vi "Kaelus PIM Config Load Instruments.vi"(7 "Tree":refnum<vi>, 8 "error in (no error)":errorcluster, 9 "Interface":T1, 10 "Port":u16=3388, 11 "IP":string="localhost" caption="Machine Location (IP / Fully Qualified Domain Name)") -> (0 "error out":errorcluster, 2 "Populated Configurations":T2[](array[typedef]) {"Calibration Date" format="%.2f"; "Parameters"."TX2pmax" format="%.1f"; "Parameters"."TX1pmax" format="%.1f"; "Parameters"."RXstop" format="%.1f"; "Parameters"."RXstart" format="%.1f"; "Parameters"."TX2stop" format="%.1f"; "Parameters"."TX2start" format="%.1f"; "Parameters"."TX1stop" format="%.1f"; "Parameters"."TX1start" format="%.1f"})   [LabVIEW 2011]
uses:
  PIM Configuration.ctl
  PIM Interface Language.ctl
  TypeDefs/Kaelus PIM PIMHW Connection CMDS.ctl
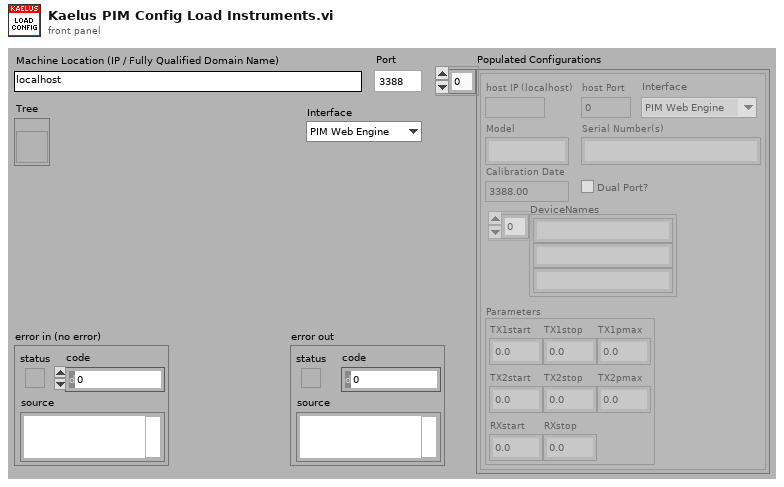
[diagram p1: front panel]
types:
  T1 = typedef "PIM Interface Language.ctl" = enum16{"PIM Web Engine", "PIM HW Engine"}
  T2 = typedef "PIM Configuration.ctl" = cluster{"host IP (localhost)":string, "host Port":u16, "Model":string, "Serial Number(s)":string, "Calibration Date":dbl, "Dual Port?":bool, "DeviceNames":string[], "Parameters":cluster{"TX1start":dbl, "TX1stop":dbl, "TX1pmax":dbl, "TX2start":dbl, "TX2stop":dbl, "TX2pmax":dbl, "RXstart":dbl, "RXstop":dbl}, "Interface":T1}
  T3 = typedef "Kaelus PIM PIMHW Connection CMDS.ctl" = enum16{"CONNECT", "DISCONNECT", "KEEP_ALIVE"}
  T4 = typedef "Test Set Definition.ctl" = cluster{"General":cluster{"ID":u32, "Model":string, "Dual Port?":bool, "Options":string, "Options":cluster{"E":bool, "K":bool, "H":bool, "W":bool, "F":bool}, "Cal File":path}, "Receiver":cluster{"Fstart, MHz":dbl, "Fstop MHz":dbl, "Fstep MHz":dbl, "IF, MHz":dbl}, "RX Band":cluster{"Fstart, MHz":dbl, "Fstop MHz":dbl}, "TX 1":cluster{"Fstart, MHz":dbl, "Fstop MHz":dbl, "Pmax, dBm":dbl, "Pstep, dB":dbl}, "TX 2":cluster{"Fstart, MHz":dbl, "Fstop MHz":dbl, "Pmax, dBm":dbl, "Pstep, dB":dbl}, "Low-side?":bool}
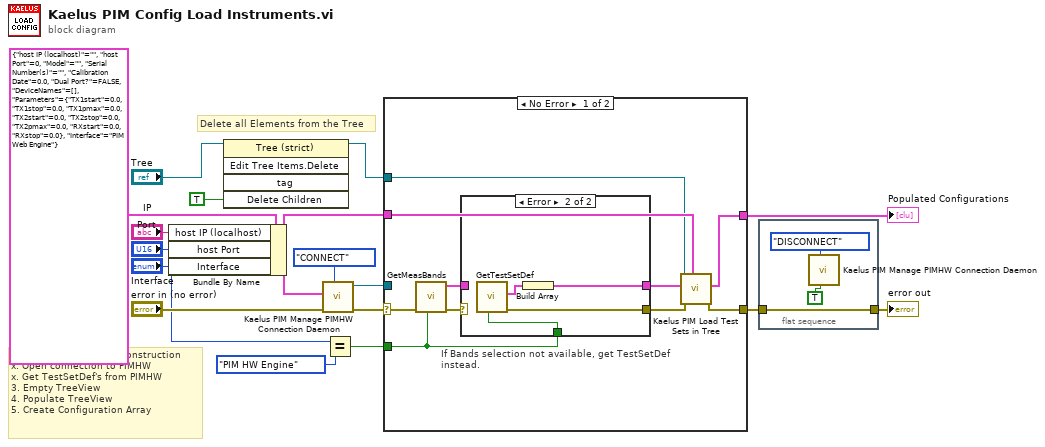
[diagram p0: block diagram]
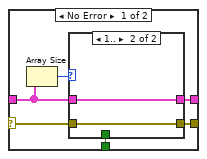
[diagram p2: hidden frame]
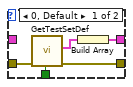
[diagram p3: hidden frame]
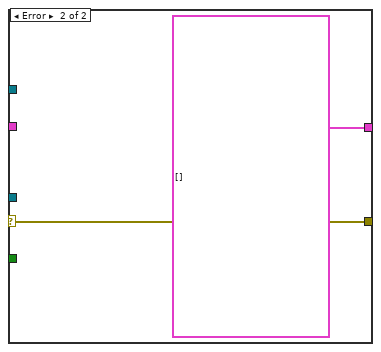
[diagram p4: hidden frame]
diagram:
  # "Delete all Elements from the Tree"
  # "x. Begin Configuration Construction\nx. Open connection to PIMHW\nx. Get TestSetDef's from PIMHW\n3. Empty TreeView\n4. Populate TreeView\n5. Create Configuration Array"
  n1 = Bundle By Name(cluster=T2 {"host IP (localhost)"="", "host Port"=0, "Model"="", "Serial Number(s)"="", "Calibration Date"=0.0, "Dual Port?"=FALSE, "DeviceNames"=[], "Parameters"={"TX1start"=0.0, "TX1stop"=0.0, "TX1pmax"=0.0, "TX2start"=0.0, "TX2stop"=0.0, "TX2pmax"=0.0, "RXstart"=0.0, "RXstop"=0.0}, "Interface"=enum."PIM Web Engine"} ("PIM Configuration"), "host IP (localhost)"="IP", "host Port"="Port", "Interface"="Interface") -> (w10:T2)
  n2 = invoke class="Tree (strict)" method="Edit Tree Items.Delete"(reference="Tree", "Delete Children"=TRUE ("Delete Children?")) -> (reference out=w7:refnum<vi>)  [unwired: 3 in, 4 out]
  n3 = call "Kaelus PIM Manage PIMHW Connection Daemon.vi"("Session Conn Cmd"=Kaelus_PIM_PIMHW_Connection_CMDS."CONNECT", "error in (no error)"="error in (no error)", "PIM Config (Connection only)"=w10) -> ("error out"=w12:errorcluster, "daemon ref out"=w13:refnum<vi>)  [unwired: 2 in, 5 out]
  n4 = Equal?(x="Interface", y=PIM_Interface_Language."PIM HW Engine" ("Interface")) -> (x = y?=w2:bool)
  n5 = case shown="No Error" w12 {
    selector: w12 -> [w27 w46]
    tunnel: w13 -> [_ _]
    tunnel: [w19 w46] -> w5
    tunnel: w7 -> [w23 _]
    tunnel: w10 -> [w24 _]
    tunnel: [w20 T2[] [] ("Populated Configurations")] -> w9
    tunnel: w2 -> [w18 _]
    frame No Error {
      n6 = call "GetMeasBands.vi"("Legacy (f)?"=w18, "error in (no error)"=w27) -> ("error out"=w26:errorcluster, "TestSets"=w25:T4[])  [unwired: 8 out]
      n7 = case "If Bands selection not available, get TestSetDef instead." shown="Error" w26 {
        selector: w26 -> [w33 _]
        tunnel: [w29 w44] -> w21
        tunnel: [w30 w43] -> w22
        tunnel: w25 -> [w31 _]
        tunnel: w18 -> [w28 w41]
        frame No Error {
          n8 = Array Size(array=w31) -> (size(s)=w32:i32)
          n9 = case shown="1.." w32 {
            tunnel: w33 -> [w37 w39]
            tunnel: w31 -> [_ w40]
            tunnel: [w35 w40] -> w30
            tunnel: [w36 w39] -> w29
            tunnel: w28 -> [w34 _]
            frame 0, Default {
              n10 = call "GetTestSetDef.vi"("Legacy (f)?"=w34, "error in (no error)"=w37) -> ("error out"=w36:errorcluster, "TestSetDef"=w38:T4)  [unwired: 8 in]
              n11 = Build Array(w38) -> (w35:T4[])
            }
            frame 1.. {
            }
          }
        }
        frame Error {
          n12 = call "GetTestSetDef.vi"("Legacy (f)?"=w41) -> ("error out"=w44:errorcluster, "TestSetDef"=w42:T4)  [unwired: 9 in]
          n13 = Build Array(w42) -> (w43:T4[])
        }
      }
      n14 = call "Kaelus PIM Load Test Sets in Tree.vi"("Base Configuration"=w24, "error in (no error)"=w21, "TestSet Definitions"=w22, "Tree Control Reference"=w23) -> ("error out"=w19:errorcluster, "Populated Configurations"=w20:T2[])  [unwired: 6 in]
    }
    frame Error {
    }
  }
  "Populated Configurations" <- w9
  n15 = flat-sequence {
    tunnel: w5 -> [w47]
    tunnel: [w47] -> w4
    frame #0 {
      n16 = call "Kaelus PIM Manage PIMHW Connection Daemon.vi"("Disconnect TCP? (f)"=TRUE, "Session Conn Cmd"=Kaelus_PIM_PIMHW_Connection_CMDS."DISCONNECT") -> ()  [unwired: 3 in, 7 out]
    }
  }
  "error out" <- w4
